vi "Open Comport.vi"(0 "Comport":refnum<visa-resource-name>, 11 "error in (no error)":errorcluster, 13 "Reply timeout (300 ms)":u32=300) -> (4 "VISA resource name out":refnum<visa-resource-name>, 15 "error out":errorcluster)   [LabVIEW 2011]
doc: "Opner comporten med den valgte VISA ingangen, om error in, gjøre ingenting"
uses:
  <vilib>/Instr/_visa.llb/VISA Configure Serial Port (Instr).vi
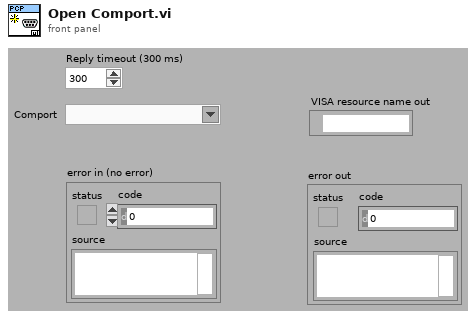
[diagram p1: front panel]
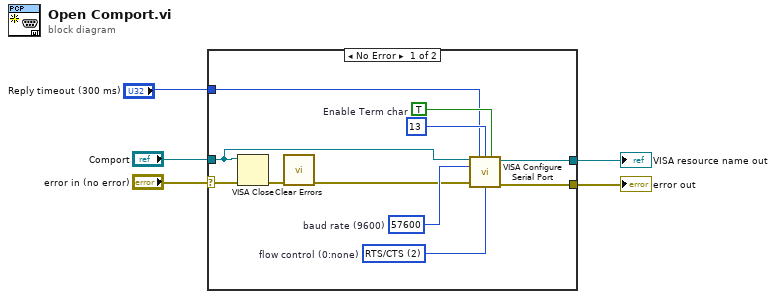
[diagram p0: block diagram]
diagram:
  n1 = case shown="No Error" "error in (no error)" {
    selector: "error in (no error)" -> [w10 w17]
    tunnel: [w14 w18] -> w5
    tunnel: [w13 w17] -> w4
    tunnel: "Comport" -> [w7 w18]
    tunnel: "Reply timeout (300 ms)" -> [w6 _]
    frame No Error {
      w15 = TRUE  # Enable Term char
      w12 = u16 2 items=["None", "XON/XOFF", "RTS/CTS", "XON/XOFF & RTS/CTS", "DTR/DSR", "XON/XOFF & DTR/DSR"]  # flow control (0:none)
      w11 = u32 57600  # baud rate (9600)
      n2 = VISA Close(VISA resource name=w7, error in (no error)=w10) -> (error out=w9:errorcluster)
      n3 = call <vilib>:"Clear Errors.vi"("error in (no error)"=w9) -> ("error out"=w8:errorcluster)  [unwired: 6 in]
      n4 = call-poly "VISA Configure Serial Port"("VISA resource name"=w7, "timeout (10sec)"=w6, "termination char\n(0xA = '\\n' = LF)"=u8 13 ("termination char\n(0xA = '\\n' = LF)"), "Enable Termination\nChar (T)"=w15, "baud rate (9600)"=w11, "error in (no error)"=w8, "flow control (0:none)"=w12) -> ("VISA resource name out"=w14:refnum<visa-resource-name>, "error out"=w13:errorcluster)  [unwired: 7 in]
    }
    frame Error {
    }
  }
  "VISA resource name out" <- w5
  "error out" <- w4
